vi "SH_savePaths.vi"(8 "error in (no error)":errorcluster, 9 "Number of Channels":i32=22, 10 "Paths":cluster{"Training Data":path}, 11 "ShapeletClass in":refnum<class "Shapelets Search Brute Force.lvclass">) -> (0 "error out":errorcluster, 3 "ShapeletClass out":refnum<class "Shapelets Search Brute Force.lvclass">)   [LabVIEW 2016, in "Shapelets Search (Brute Force).lvlib" / "Shapelets Search Brute Force.lvclass"]
uses:
  Shapelets Search Brute Force.lvclass
  Shapelets Search Brute Force.lvclass/Shapelets Search Brute Force.ctl
panel:
  # "This VI is a part of BCI Design library, http://www.ru-bci.org \nCopyright © 2020, Sotnikov Peter, All rights reserved. License: GNU GPLv3"
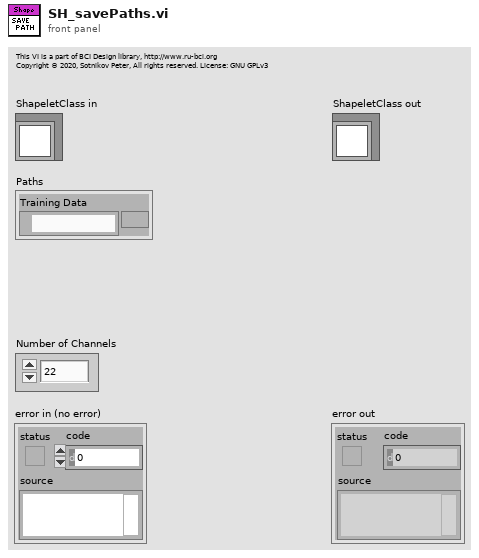
[diagram p1: front panel]
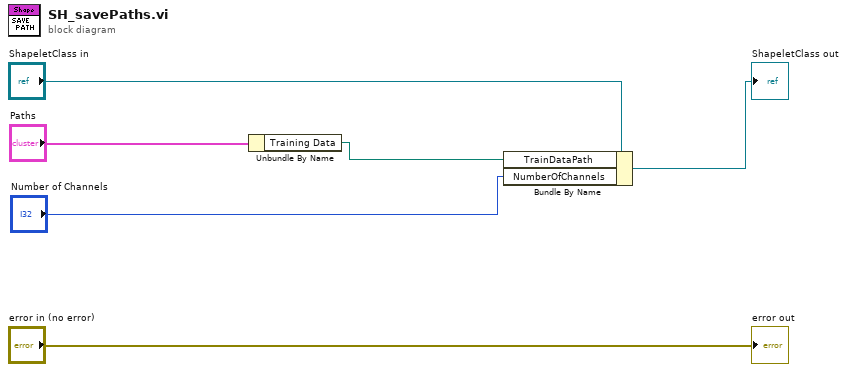
[diagram p0: block diagram]
diagram:
  n1 = Unbundle By Name("Paths") -> ("Training Data"=w1:path)
  n2 = Bundle By Name(cluster="ShapeletClass in", "TrainDataPath"=w1, "NumberOfChannels"="Number of Channels") -> (→"ShapeletClass out":refnum<class "Shapelets Search Brute Force.lvclass">)
  "error out" <- "error in (no error)"
